vi "Print.vi"(1 "String":string) -> ()   [LabVIEW 2014, in "Raspberry Pi Compatible Compiler for LabVIEW.lvlib" / "Console.lvlib"]
doc: "Passes the value of String to stdout. Primarily intended for console applications it can also be used for debugging GUI applications."
uses:
  Console.lvlib
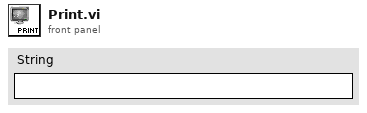
[diagram p1: front panel]
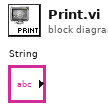
[diagram p0: block diagram]
diagram:
